vi "Write XboxJoysticks.vi"(8 "error in (no error)":errorcluster, 10 "XboxJoysticks":T1 {"RightJoystick"."Right" scale=-1.0..1.0; "RightJoystick"."Forward" scale=-1.0..1.0; "LeftJoystick"."Right" scale=-1.0..1.0; "LeftJoystick"."Forward" scale=-1.0..1.0}, 11 "XBoxController in":refnum<class "XBoxController.lvclass">) -> (0 "error out":errorcluster, 3 "XBoxController out":refnum<class "XBoxController.lvclass">)   [LabVIEW 2013, in "XBoxController.lvlib" / "XBoxController.lvclass"]
uses:
  XBoxController.lvclass
  XboxJoysticks.ctl
  XBoxController.lvclass/XBoxController.ctl
  XBoxController.lvlib
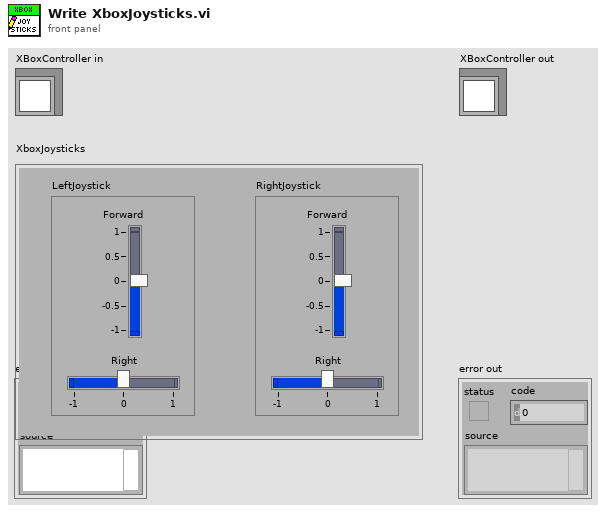
[diagram p1: front panel]
types:
  T1 = typedef "XBoxController.lvlib/XboxJoysticks.ctl" = cluster{"LeftJoystick":cluster{"Forward":dbl, "Right":dbl}, "RightJoystick":cluster{"Forward":dbl, "Right":dbl}}
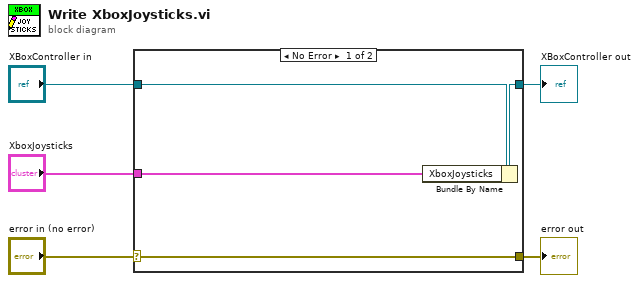
[diagram p0: block diagram]
diagram:
  n1 = case shown="No Error" "error in (no error)" {
    selector: "error in (no error)" -> [w9 w10]
    tunnel: [w9 w10] -> w4
    tunnel: [w7 w11] -> w2
    tunnel: "XBoxController in" -> [w8 w11]
    tunnel: "XboxJoysticks" -> [w6 _]
    frame No Error {
      n2 = Bundle By Name(cluster=w8, "XboxJoysticks"=w6) -> (w7:refnum<class "XBoxController.lvclass">)
    }
    frame Error {
    }
  }
  "error out" <- w4
  "XBoxController out" <- w2
